vi "encodeStream.vi"(8 "error in (no error)":errorcluster, 11 "tBSONArray in":refnum<class "tBSONArray.lvclass">) -> (0 "error out":errorcluster, 2 "Byte Array":u8[](array[numeric]), 3 "tBSONArray out":refnum<class "tBSONArray.lvclass">)   [LabVIEW 2013, in "BSON.lvlib" / "tBSONArray.lvclass"]
uses:
  tBSONArray.lvclass
  tBSONDocument/tBSONDocument.lvclass
  tBSONElement/tBSONElement.lvclass
  getValue.vi
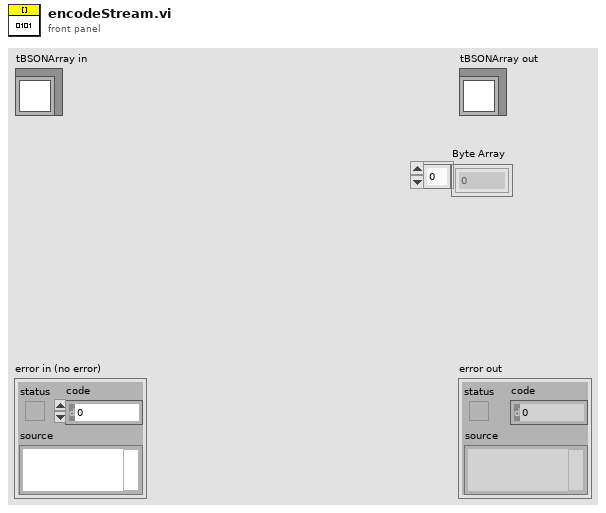
[diagram p1: front panel]
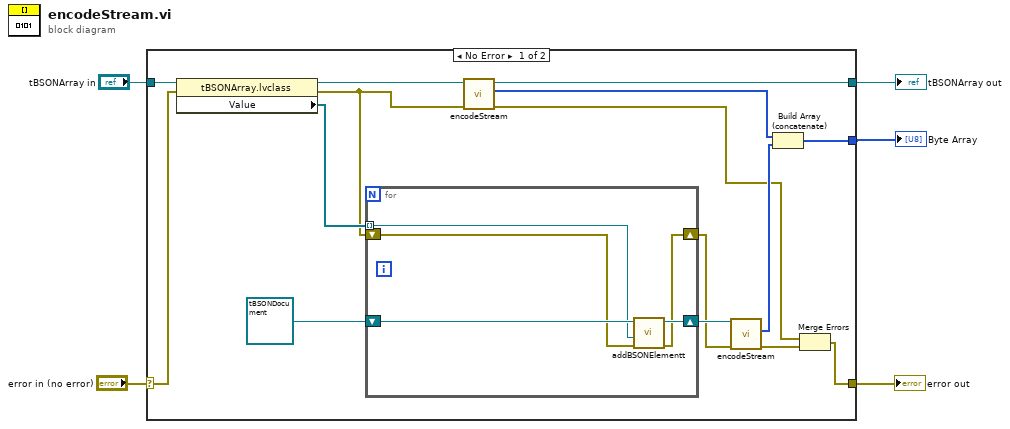
[diagram p0: block diagram]
diagram:
  n1 = case shown="No Error" "error in (no error)" {
    selector: "error in (no error)" -> [w19 w26]
    tunnel: "tBSONArray in" -> [w20 w27]
    tunnel: [w9 w27] -> w4
    tunnel: [w11 w26] -> w3
    tunnel: [w18 _] -> w1
    frame No Error {
      n2 = property class="tBSONArray.lvclass"(reference=w20, error in=w19) -> (reference out=w10:refnum<class "tBSONArray.lvclass">, error out=w8:errorcluster, "Value"=w17:refnum<class "tBSONElement.lvclass">[])
      n3 = for {
        tunnel: w17 -> [w22] mode=indexing
        shift-right: [w23] -> w14
        shift-left: w8 -> [w21]
        shift-right: [w24] -> w15
        shift-left: refnum<class "tBSONDocument.lvclass"> refnum ("BSON.lvlib:tBSONDocument.lvclass") -> [w25]
        n4 = call "addBSONElementt.vi"("error in (no error)"=w21, "Element"=w22, "tBSONDocument in"=w25) -> ("error out"=w23:errorcluster, "tBSONDocument out"=w24:refnum<class "tBSONDocument.lvclass">)  [unwired: 7 in]
      }
      n5 = call-parent "encodeStream.vi"("error in (no error)"=w8, "tBSONElement in"=w10) -> ("error out"=w7:errorcluster, "Byte Array"=w6:u8[], "tBSONElement out"=w9:refnum<class "tBSONArray.lvclass">)  [unwired: 7 in]
      n6 = call "encodeStream.vi"("error in (no error)"=w14, "tBSONDocument in"=w15) -> ("error out"=w12:errorcluster, "Byte Data"=w13:u8[])  [unwired: 7 in, 1 out]
      n7 = Build Array (concatenate)(w6, w13) -> (w18:u8[])
      n8 = Merge Errors(w7, w12) -> (w11:errorcluster)
    }
    frame Error {
    }
  }
  "error out" <- w3
  "tBSONArray out" <- w4
  "Byte Array" <- w1
